vi "Common ini Keys.vi"(7 "Log Sinks in":refnum<class "Log Sinks.lvclass">, 8 "error in (no error)":errorcluster, 9 "section":string, 11 "refnum in":T1) -> (0 "error out":errorcluster, 3 "refnum out":T1, 5 "Log Sinks out":refnum<class "Log Sinks.lvclass">)   [LabVIEW 2019, in "TSC Event Logger.lvlib" / "Log Sinks.lvclass"]
doc: "Read the ini keys that are common for the different sink types.\n\n<b>Code Developed By:</b>\nTechnology Service Corporation\nBloomington, IN 47403\nwww.tsc.com/atcs\n\nDeveloper:\nDaniel Coons"
uses:
  Log Sinks.lvclass
  <vilib>/Utility/config.llb/NI_LVConfig.lvlib
  <vilib>/Utility/config.llb/Read Key (String).vi
  Layouts/SimpleLayout/SimpleLayout.lvclass
  Layouts/JSONLayout/JSONLayout.lvclass
  Layouts/CSVLayout/CSVLayout.lvclass
  <vilib>/Utility/config.llb/Read Key (I32).vi
  C:/Development/Open Source/tsc-event-logger/Layouts/Layout.lvclass
  <vilib>/Utility/config.llb/Config Data RefNum.ctl
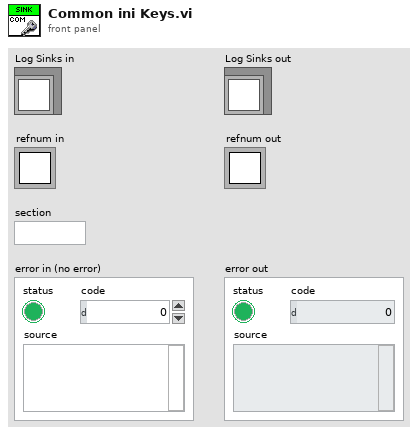
[diagram p1: front panel]
types:
  T1 = typedef "NI_LVConfig.lvlib/Config Data RefNum.ctl" = refnum<k1>
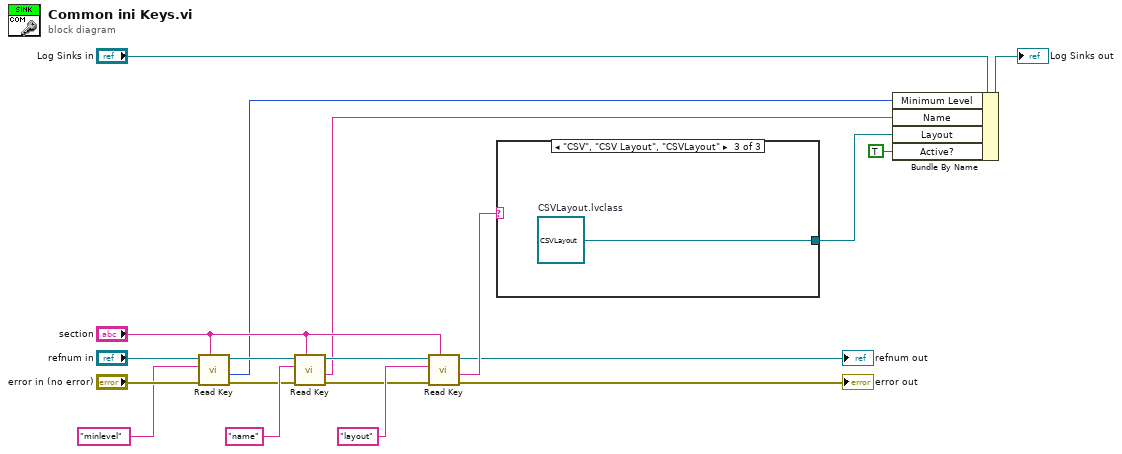
[diagram p0: block diagram]
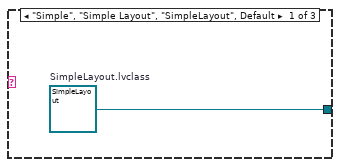
[diagram p2: hidden frame]
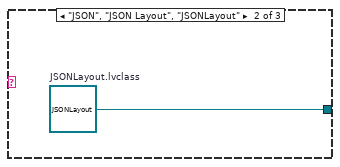
[diagram p3: hidden frame]
diagram:
  n1 = call-poly <vilib>:"Read Key.vi"("section"="section", "error in (no error)"="error in (no error)", "key"="minlevel", "refnum"="refnum in") -> ("error out"=w6:errorcluster, "value"=w4:i32, "refnum out"=w7:T1)  [unwired: 4 in, 1 out]
  n2 = call-poly <vilib>:"Read Key.vi"("section"="section", "error in (no error)"=w6, "key"="name", "refnum"=w7) -> ("error out"=w9:errorcluster, "value"=w3:string, "refnum out"=w15:T1)  [unwired: 4 in, 1 out]
  n3 = call-poly <vilib>:"Read Key.vi"("section"="section", "error in (no error)"=w9, "key"="layout", "refnum"=w15) -> ("error out"=→"error out":errorcluster, "value"=w19:string, "refnum out"=→"refnum out":T1)  [unwired: 4 in, 1 out]
  n4 = case shown="\"CSV\", \"CSV Layout\", \"CSVLayout\"" w19 {
    tunnel: [w20 w21 w22] -> w2
    frame "Simple", "Simple Layout", "SimpleLayout", Default {
      w20 = refnum<class "SimpleLayout.lvclass"> refnum  # SimpleLayout.lvclass
    }
    frame "JSON", "JSON Layout", "JSONLayout" {
      w21 = refnum<class "JSONLayout.lvclass"> refnum  # JSONLayout.lvclass
    }
    frame "CSV", "CSV Layout", "CSVLayout" {
      w22 = refnum<class "CSVLayout.lvclass"> refnum  # CSVLayout.lvclass
    }
  }
  n5 = Bundle By Name(cluster="Log Sinks in", "Minimum Level"=w4, "Name"=w3, "Layout"=w2, "Active?"=TRUE) -> (→"Log Sinks out":refnum<class "Log Sinks.lvclass">)
